vi "ForLoop_AutoIndexing.vi"() -> ()   [LabVIEW 2018]
panel:
  out "숫자형 2":i32
  out "배열":i32[](array[numeric])
  out "숫자형":i32
  out "원소":i32
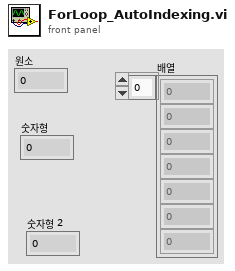
[diagram p1: front panel]
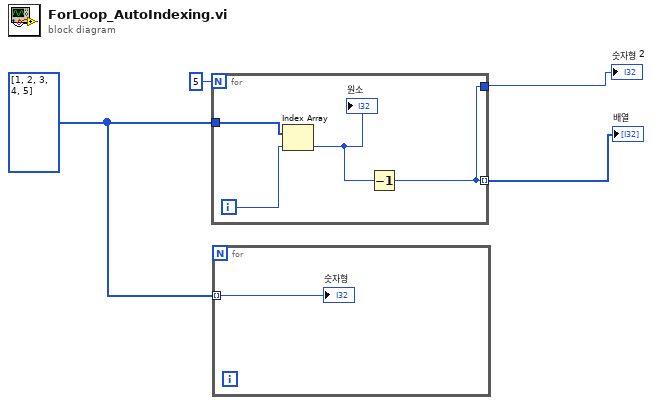
[diagram p0: block diagram]
diagram:
  w3 = i32[] [1, 2, 3, 4, 5]
  n1 = for {
    N: 5 -> [_]
    tunnel: w3 -> [w7]
    tunnel: [w5] -> w2 mode=indexing
    tunnel: [w5] -> w1
    i -> [w8]
    n2 = Index Array(array=w7, index=w8) -> (element=w6:i32)
    "원소" <- w6
    n3 = Decrement(x=w6) -> (x-1=w5:i32)
  }
  "배열" <- w2
  "숫자형 2" <- w1
  n4 = for {
    tunnel: w3 -> [w9] mode=indexing
    "숫자형" <- w9
  }
